vi "Can Edit Cell.vi"(0 "Rows":T1[](array[typedef]), 5 "Items":i32[](array[numeric]), 7 "Cell":T3) -> (4 "item":T1, 6 "row":i32, 8 "can edit?":bool, 15 "enum?":bool)   [LabVIEW 2015, in "KPropertyTable.xctl"]
uses:
  KPropertyTable.xctl
  <vilib>/Utility/miscctls.llb/LVRowAndColumnTypeDef.ctl
  RowData.ctl
  DataType.ctl
  KTable/ColumnType.ctl
  KTable/KTable.xctl
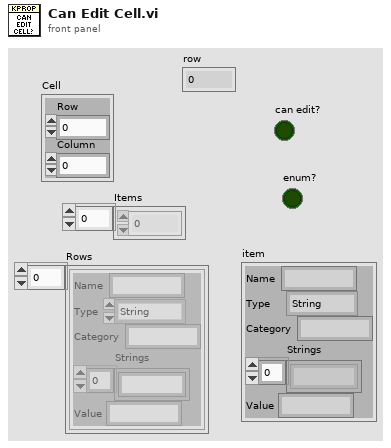
[diagram p1: front panel]
types:
  T1 = typedef "KPropertyTable.xctl/RowData.ctl" = cluster{"Name":string, "Type":T2, "Category":string, "Strings":string[], "Value":string}
  T2 = typedef "KPropertyTable.xctl/DataType.ctl" = enum16{"String", "Enum", "Int", "Double", "Boolean", "Ring", "Formula"}
  T3 = typedef "LVRowAndColumnTypeDef.ctl" = cluster{"Row":i32, "Column":i32}
  T4 = typedef "KTable.xctl/ColumnType.ctl" = enum16{"String", "Enum", "Int", "Double", "Boolean", "Ring", "Formula", "Color"}
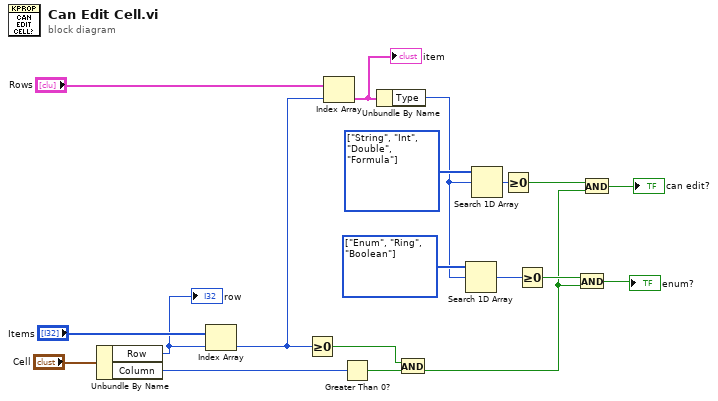
[diagram p0: block diagram]
diagram:
  w6 = T2[] [enum."String", enum."Int", enum."Double", enum."Formula"] items=["String", "Enum", "Int", "Double", "Boolean", "Ring", "Formula"] ("y")
  w18 = T4[] [enum."Enum", enum."Ring", enum."Boolean"] items=["String", "Enum", "Int", "Double", "Boolean", "Ring", "Formula", "Color"] ("y")
  n1 = Unbundle By Name("Cell") -> ("Row"=w1:i32, "Column"=w13:i32)
  "row" <- w1
  n2 = Index Array(array="Items", index=w1) -> (element=w10:i32)
  n3 = Greater Or Equal To 0?(x=w10) -> (x >= 0?=w9:bool)
  n4 = Index Array(array="Rows", index=w10) -> (element=w19:T1)
  "item" <- w19
  n5 = Greater Than 0?(x=w13) -> (x > 0?=w15:bool)
  n6 = Unbundle By Name(w19) -> ("Type"=w5:T2)
  n7 = And(x=w9, y=w15) -> (x .and. y?=w3:bool)
  n8 = Search 1D Array(1D array=w18, element=w5) -> (index of element=w17:i32)  [unwired: 1 in]
  n9 = Search 1D Array(1D array=w6, element=w5) -> (index of element=w7:i32)  [unwired: 1 in]
  n10 = Greater Or Equal To 0?(x=w7) -> (x >= 0?=w4:bool)
  n11 = Greater Or Equal To 0?(x=w17) -> (x >= 0?=w16:bool)
  n12 = And(x=w16, y=w3) -> (x .and. y?=→"enum?":bool)
  n13 = And(x=w4, y=w3) -> (x .and. y?=→"can edit?":bool)
